vi "SRDG535.PC Get Output.vi"(0 "i ref in":refnum<vi>, 4 "Channel":T2 items=["T0", "A", "B", "AB", "C", "D", "CD"], 5 "error IO":errorcluster) -> (14 "i ref out":refnum<vi>, 19 "error out":errorcluster)   [LabVIEW 2014, in "SRDG535.lvlib"]
doc: "This VI communicates with the hardware."
uses:
  SRDG535.lvlib
  SRDG535.Channel.ctl
  SRDG535.Channel Output.ctl
  instr.lib/SRDG535/Stanford Research DG535 - Driver np.lvlib
  CS_PHELIX/PH_Basics/PH_Common/PH_Common.lvlib
panel:
  in  "Output":T1 {"Mode" items=["TTL", "NIM", "ECL", "VAR"]; "Offset (V)" min=-3.0 max=4.0 format="%.2f"; "Amplitude (V)" min=-3.0 max=4.0 format="%.2f"}
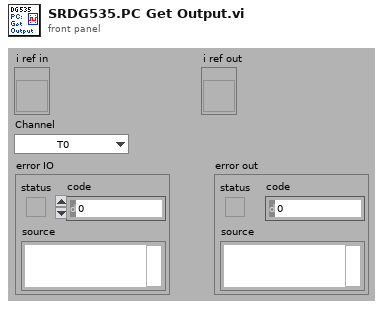
[diagram p1: front panel]
types:
  T1 = typedef "SRDG535.lvlib/SRDG535.Channel Output.ctl" = cluster{"Inversion":bool, "Amplitude (V)":dbl, "Offset (V)":dbl, "Mode":i32, "Load":bool}
  T2 = typedef "SRDG535.lvlib/SRDG535.Channel.ctl" = u16
  T3 = typedef "SRDG535.lvlib/SRDG535.i attribute.ctl" = cluster{"GPIB address":string, "Device error":errorcluster, "GUI Refs":cluster{"Delete":refnum<vi>, "Device Error":refnum<vi>, "Information":refnum<vi>, "Output":refnum<vi>, "Delay":refnum<vi>, "Trigger":refnum<vi>}, "Output Settings":T4, "Service ID Rate":i32, "Service IDs Channelinfo":i32[], "Delay Settings":T5, "Trigger Settings":T6}
  T4 = typedef "SRDG535.lvlib/SRDG535.Output.ctl" = cluster{"CH T0":T1, "CH A":T1, "CH B":T1, "CH AB":T1, "CH C":T1, "CH D":T1, "CH CD":T1}
  T5 = typedef "SRDG535.lvlib/SRDG535.Delay.ctl" = cluster{"CH A":cluster{"rel to":u32, "Delay (s)":dbl}, "CH B":cluster{"rel to":u32, "Delay (s)":dbl}, "CH C":cluster{"rel to":u32, "Delay (s)":dbl}, "CH D":cluster{"rel to":u32, "Delay (s)":dbl}}
  T6 = typedef "SRDG535.lvlib/SRDG535.Trigger.ctl" = cluster{"trigger":u32, "Impedance":bool, "Slope":bool, "burst count":i32, "external level (V)":sgl, "Internal/Burst Rate (Hz)":dbl, "Burst Period":i32}
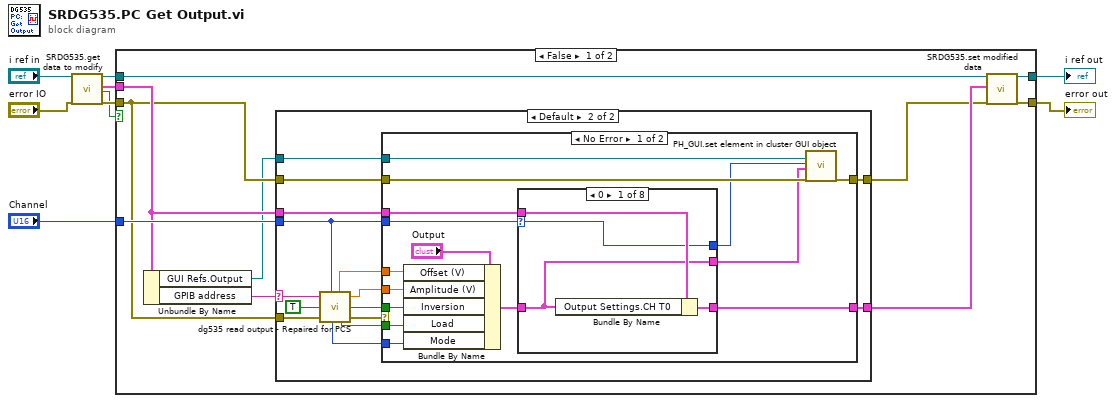
[diagram p0: block diagram]
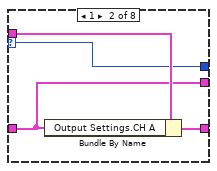
[diagram p3: hidden frame]
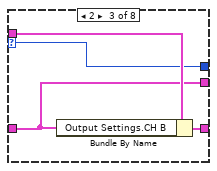
[diagram p4: hidden frame]
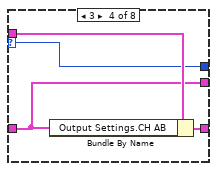
[diagram p5: hidden frame]
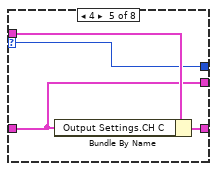
[diagram p6: hidden frame]
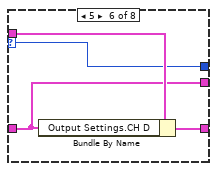
[diagram p7: hidden frame]
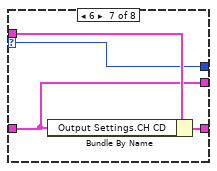
[diagram p8: hidden frame]
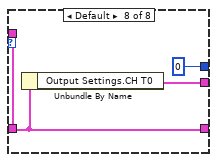
[diagram p9: hidden frame]
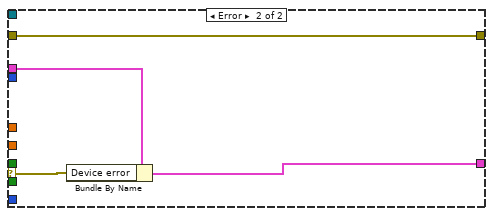
[diagram p10: hidden frame]
diagram:
  n1 = call "SRDG535.get data to modify.vi"("i ref in"="i ref in", "error in (no error)"="error IO") -> ("i ref out"=w5:refnum<vi>, "i attribute"=w9:T3, "timed out"=w2:bool, "error out"=w7:errorcluster)  [unwired: 14 in]
  n2 = case shown="False" w2 {
    tunnel: w9 -> [w14 _]
    tunnel: [w19 w87] -> w8
    tunnel: w7 -> [w12 w87]
    tunnel: [w18 w88] -> w6
    tunnel: w5 -> [w17 w88]
    tunnel: "Channel" -> [w15 _]
    frame False {
      n3 = Unbundle By Name(w14) -> ("GUI Refs.Output"=w10:refnum<vi>, "GPIB address"=w16:string)
      n4 = case shown="Default" w16 {
        selector: w16 -> [_ w34]
        tunnel: w12 -> [_ w36]
        tunnel: w15 -> [_ w25]
        tunnel: w14 -> [w21 w33]
        tunnel: [w21 w32] -> w13
        tunnel: w12 -> [w20 w24]
        tunnel: [w20 w23] -> w11
        tunnel: w10 -> [_ w22]
        frame "", "N/A" {
        }
        frame Default {
          n5 = call "dg535 read output - Repaired for PCS.vi"("GPIB address"=w34, "output"=w25, "read"=TRUE ("set"), "error in"=w36) -> ("mode"=w26:u8, "offset"=w28:dbl, "amplitude"=w29:dbl, "inversion"=w30:bool, "load"=w27:bool, "error out"=w31:errorcluster)
          n6 = case shown="No Error" w31 {
            selector: w31 -> [_ w86]
            tunnel: w33 -> [w51 w85]
            tunnel: [w50 w84] -> w32
            tunnel: w30 -> [w46 _]
            tunnel: w29 -> [w47 _]
            tunnel: w28 -> [w48 _]
            tunnel: w27 -> [w45 _]
            tunnel: w26 -> [w44 _]
            tunnel: w25 -> [w42 _]
            tunnel: w24 -> [w41 w83]
            tunnel: [w40 w83] -> w23
            tunnel: w22 -> [w39 _]
            frame No Error {
              n7 = Bundle By Name(cluster="Output", "Offset (V)"=w48, "Amplitude (V)"=w47, "Inversion"=w46, "Load"=w45, "Mode"=w44) -> (w43:T1)
              n8 = case shown="0" w42 {
                selector: w42 -> [w52 w56 w60 w64 w68 w72 w76 _]
                tunnel: w51 -> [w55 w59 w63 w67 w71 w75 w79 w81]
                tunnel: [w54 w58 w62 w66 w70 w74 w78 w81] -> w50
                tunnel: w43 -> [w53 w57 w61 w65 w69 w73 w77 _]
                tunnel: [w53 w57 w61 w65 w69 w73 w77 w80] -> w38
                tunnel: [w52 w56 w60 w64 w68 w72 w76 0] -> w37
                frame 0 {
                  n9 = Bundle By Name(cluster=w55, "Output Settings.CH T0"=w53) -> (w54:T3)
                }
                frame 1 {
                  n10 = Bundle By Name(cluster=w59, "Output Settings.CH A"=w57) -> (w58:T3)
                }
                frame 2 {
                  n11 = Bundle By Name(cluster=w63, "Output Settings.CH B"=w61) -> (w62:T3)
                }
                frame 3 {
                  n12 = Bundle By Name(cluster=w67, "Output Settings.CH AB"=w65) -> (w66:T3)
                }
                frame 4 {
                  n13 = Bundle By Name(cluster=w71, "Output Settings.CH C"=w69) -> (w70:T3)
                }
                frame 5 {
                  n14 = Bundle By Name(cluster=w75, "Output Settings.CH D"=w73) -> (w74:T3)
                }
                frame 6 {
                  n15 = Bundle By Name(cluster=w79, "Output Settings.CH CD"=w77) -> (w78:T3)
                }
                frame Default {
                  n16 = Unbundle By Name(w81) -> ("Output Settings.CH T0"=w80:T1)
                }
              }
              n17 = call "PH_GUI.set element in cluster GUI object.vi"("Cluster Ref"=w39, "Cluster index"=w37, "Value"=w38, "error in (no error)"=w41) -> ("error out"=w40:errorcluster)  [unwired: 15 in]
            }
            frame Error {
              n18 = Bundle By Name(cluster=w85, "Device error"=w86) -> (w84:T3)
            }
          }
        }
      }
      n19 = call "SRDG535.set modified data.vi"("i ref in"=w17, "i attribute"=w13, "error in (no error)"=w11) -> ("i ref out"=w18:refnum<vi>, "error out"=w19:errorcluster)  [unwired: 15 in]
    }
    frame True {
    }
  }
  "error out" <- w8
  "i ref out" <- w6
